vi "Get Target ref.vi"(8 "error in (no error)":errorcluster, 10 "Target Name":string, 11 "Project in":refnum<vi>) -> (0 "error out":errorcluster, 2 "Target ref out":refnum<vi>, 3 "Project out":refnum<vi>)   [LabVIEW 2019, in "gRPC Scripting Tools.lvlib"]
uses:
  gRPC Scripting Tools.lvlib
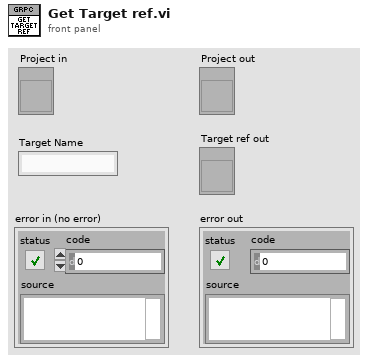
[diagram p1: front panel]
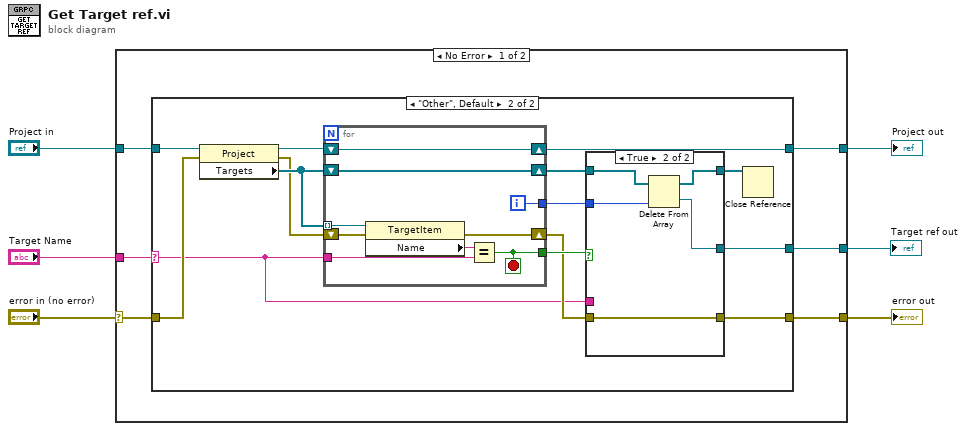
[diagram p0: block diagram]
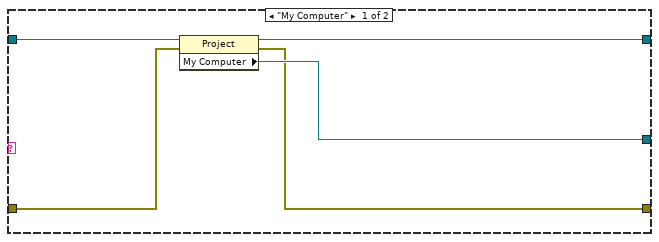
[diagram p2: hidden frame]
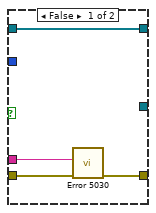
[diagram p3: hidden frame]
diagram:
  n1 = case shown="No Error" "error in (no error)" {
    selector: "error in (no error)" -> [w8 w50]
    tunnel: [w10 w51] -> w6
    tunnel: [w7 w50] -> w5
    tunnel: "Project in" -> [w12 w51]
    tunnel: "Target Name" -> [w11 _]
    tunnel: [w9 _] -> w1
    frame No Error {
      n2 = case shown="\"Other\", Default" w11 {
        selector: w11 -> [_ w18]
        tunnel: w12 -> [w17 w31]
        tunnel: [w16 w29] -> w10
        tunnel: [w15 w20] -> w9
        tunnel: w8 -> [w14 w27]
        tunnel: [w13 w19] -> w7
        frame "My Computer" {
          n3 = property class="Project"(reference=w17, error in=w14) -> (reference out=w16:refnum<vi>, error out=w13:errorcluster, "My Computer"=w15:refnum<vi>)
        }
        frame "Other", Default {
          n4 = property class="Project"(reference=w31, error in=w27) -> (reference out=w30:refnum<vi>, error out=w26:errorcluster, "Targets"=w28:refnum<vi>[])
          n5 = for {
            tunnel: w28 -> [w49] mode=indexing
            shift-right: [w48] -> w29
            shift-left: w30 -> [w48]
            tunnel: w18 -> [w41]
            shift-right: [w45] -> w24
            shift-left: w28 -> [w45]
            shift-right: [w42] -> w22
            shift-left: w26 -> [w46]
            tunnel: [w44] -> w25
            tunnel: [w43] -> w23
            i -> [w43]
            stop <- w44 stop-if-true
            n6 = property class="TargetItem"(reference=w49, error in=w46) -> (error out=w42:errorcluster, "Name"=w47:string)  [unwired: 1 out]
            n7 = Equal?(x=w47, y=w41) -> (x = y?=w44:bool)
          }
          n8 = case shown="True" w25 {
            tunnel: w24 -> [w35 w40]
            tunnel: w23 -> [_ w39]
            tunnel: [w35 w38] -> w21
            tunnel: w22 -> [w34 w36]
            tunnel: [_ w37] -> w20
            tunnel: [w33 w36] -> w19
            tunnel: w18 -> [w32 _]
            frame False {
              n9 = call "Error 5030.vi"("error in (no error)"=w34, "Target Name"=w32) -> ("error out"=w33:errorcluster)  [unwired: 9 in]
            }
            frame True {
              n10 = Delete From Array(array=w40, index=w39) -> (deleted portion=w37:refnum<vi>, array with subset deleted=w38:refnum<vi>[])  [unwired: 1 in]
            }
          }
          n11 = Close Reference(reference=w21) -> ()  [unwired: 1 in, 1 out]
        }
      }
    }
    frame Error {
    }
  }
  "Project out" <- w6
  "error out" <- w5
  "Target ref out" <- w1
